vi "Get Number 5 Digit 5.vi"(10 "Pattern Number 6":string, 11 "Array":string[][](array[string])) -> (2 "Pattern number 5":string, 3 "Digit 5":string)   [LabVIEW 2019, in "Day 8.lvlib"]
uses:
  Day 8.lvlib
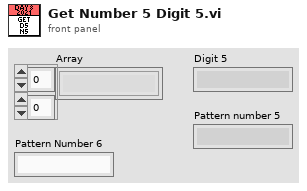
[diagram p1: front panel]
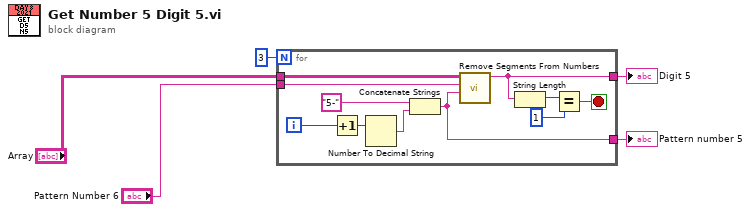
[diagram p0: block diagram]
diagram:
  n1 = for {
    N: 3 -> [_]
    tunnel: "Array" -> [w16]
    tunnel: [w6] -> w3
    tunnel: [w11] -> w4
    tunnel: "Pattern Number 6" -> [w10]
    i -> [w12]
    stop <- w7 stop-if-true
    n2 = Increment(x=w12) -> (x+1=w13:i32)
    n3 = Number To Decimal String(number=w13) -> (decimal integer string=w14:string)  [unwired: 1 in]
    n4 = Concatenate Strings("5-" ("Pattern For Number Of Letters A"), w14) -> (w11:string)
    n5 = call "Remove Segments From Numbers.vi"("Pattern For Letter Of Letters B"=w11, "Pattern For Number Of Letters A"=w10, "Array"=w16) -> ("Result"=w6:string)  [unwired: 8 in]
    n6 = String Length(string=w6) -> (length=w9:i32)
    n7 = Equal?(x=w9, y=1) -> (x = y?=w7:bool)
  }
  "Pattern number 5" <- w4
  "Digit 5" <- w3
